vi "Forward Auto V.3.0.vi"(8 "Desired Angle":dbl, 11 "Encoder Distance (in.)":dbl) -> (3 "Stop":bool)   [LabVIEW 2017]
uses:
  Robot Global Data V.3.0.vi
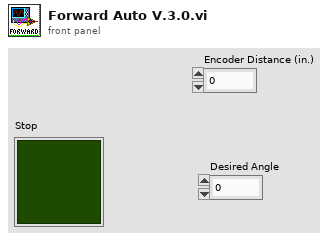
[diagram p1: front panel]
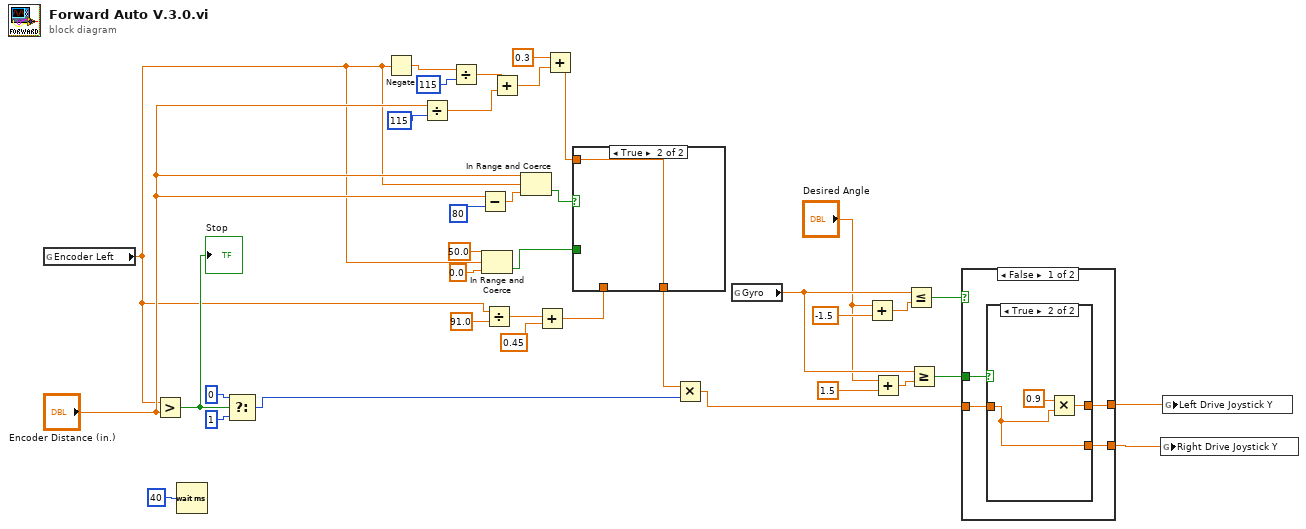
[diagram p0: block diagram]
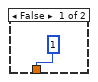
[diagram p3: hidden frame]
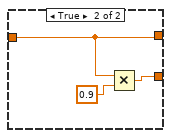
[diagram p5: hidden frame]
diagram:
  n1 = global read "Robot Global Data V.3.0.vi" "Encoder Left"() -> (w18:dbl)
  n2 = Greater?(x=w18, y="Encoder Distance (in.)") -> (0:w35:bool)
  "Stop" <- w35
  n3 = Wait (ms)(milliseconds to wait=u32 40) -> ()  [unwired: 1 out]
  n4 = Select(t=0, s=w35, f=1) -> (s? t:f=w33:i32)
  n5 = Negate(x=w18) -> (-x=w31:dbl)
  n6 = Divide(x="Encoder Distance (in.)", y=115) -> (x/y=w29:dbl)
  n7 = Divide(x=w31, y=115) -> (x/y=w28:dbl)
  n8 = Subtract(x="Encoder Distance (in.)", y=80) -> (x-y=w25:dbl)
  n9 = In Range and Coerce(upper limit=50.0, x=w18, lower limit=0.0) -> (In Range?=w19:bool)  [unwired: 1 out]
  n10 = Divide(x=w18, y=91.0) -> (x/y=w16:dbl)
  n11 = Add(x=w28, y=w29) -> (x+y=w13:dbl)
  n12 = In Range and Coerce(upper limit="Encoder Distance (in.)", x=w18, lower limit=w25) -> (In Range?=w24:bool)  [unwired: 1 out]
  n13 = Add(x=w16, y=0.45) -> (x+y=w14:dbl)
  n14 = Add(x=0.3, y=w13) -> (x+y=w11:dbl)
  n15 = case shown="True" w24 {
    tunnel: w11 -> [_ w43]
    tunnel: [w39 w43] -> w23
    tunnel: w19 -> [w40 _]
    tunnel: w14 -> [w38 _]
    frame False {
      n16 = case shown="True" w40 {
        tunnel: [1 w42] -> w39
        tunnel: w38 -> [_ w42]
        frame False {
        }
        frame True {
        }
      }
    }
    frame True {
    }
  }
  n17 = Multiply(x=w23, y=w33) -> (x*y=w32:dbl)
  n18 = global read "Robot Global Data V.3.0.vi" "Gyro"() -> (w10:dbl)
  n19 = Add(x="Desired Angle", y=-1.5) -> (x+y=w8:dbl)
  n20 = Add(x="Desired Angle", y=1.5) -> (x+y=w7:dbl)
  n21 = Less Or Equal?(x=w10, y=w8) -> (x <= y?=w4:bool)
  n22 = Greater Or Equal?(x=w10, y=w7) -> (x >= y?=w3:bool)
  n23 = case shown="False" w4 {
    tunnel: [w45 w54] -> w1
    tunnel: [w46 w53] -> w2
    tunnel: w32 -> [w47 w54]
    tunnel: w3 -> [w44 _]
    frame False {
      n24 = case shown="True" w44 {
        tunnel: w47 -> [w48 w51]
        tunnel: [w48 w51] -> w46
        tunnel: [w48 w50] -> w45
        frame False {
        }
        frame True {
          n25 = Multiply(x=0.9, y=w51) -> (x*y=w50:dbl)
        }
      }
    }
    frame True {
      n26 = Multiply(x=w54, y=0.9) -> (x*y=w53:dbl)
    }
  }
  n27 = global write "Robot Global Data V.3.0.vi" "Right Drive Joystick Y"(w2) -> ()
  n28 = global write "Robot Global Data V.3.0.vi" "Left Drive Joystick Y"(w1) -> ()
